vi "Test Zip Methods.vi"() -> ()   [LabVIEW 2016]
uses:
  <userlib>/_OpenG.lib/file/file.llb/Build Path - File Names Array__ogtk.vi
panel:
  out "Numeric":i32=241
  in  "Method":enum16{"MGI", "G", "LV", "7z"}(ring)=enum."7z"
  in  "Table Control":string[][](table)=[["Method", "Size (B)", "Time (s)", "Notes"], ["MGI", "15828699", "20.5822", "Sometimes Errors?"], ["G", "15839557", "5.54458", "Easy to use"], ["LV", "15839557", "4.38332", "Paths cumbersome"], ["7zip", "11000000", "long", "super cumbersome"]]
  out "time (s)":dbl=0.026690200000302866
  out "size (B)":i64
  in  "Root Directory":path=path "C:/user/patrick/git/LV-to-ITX/src/Tests/Example Data/ITX Folder/MNK/SA02836H.20170110/36 - Sweep B - 2"
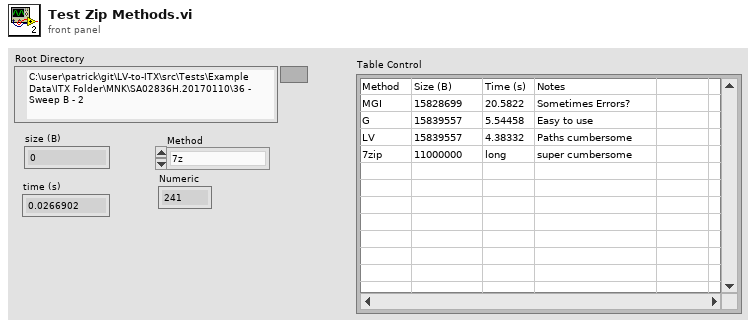
[diagram p1: front panel]
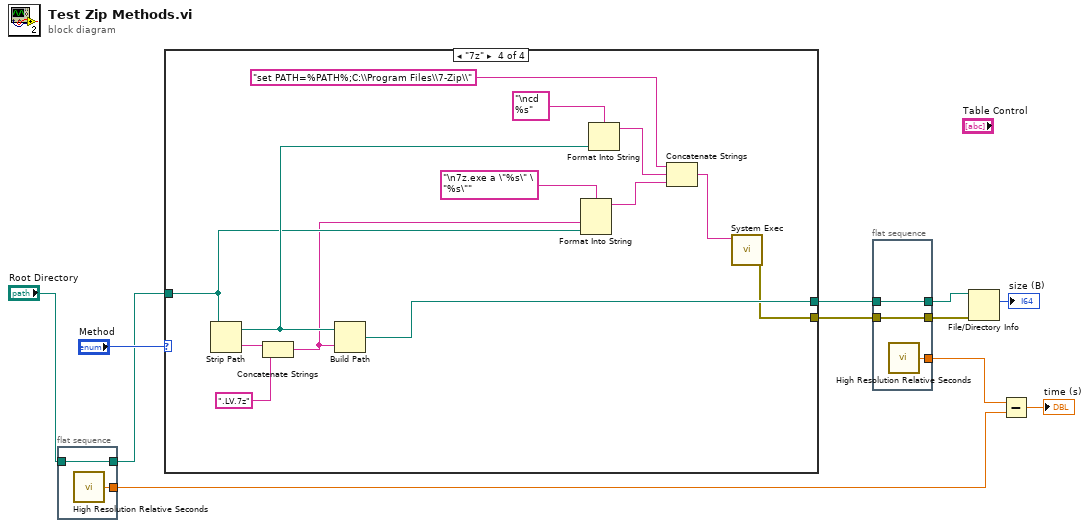
[diagram p0: block diagram]
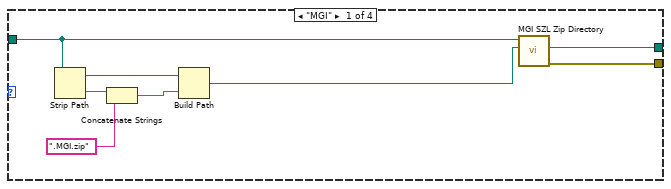
[diagram p2: hidden frame]
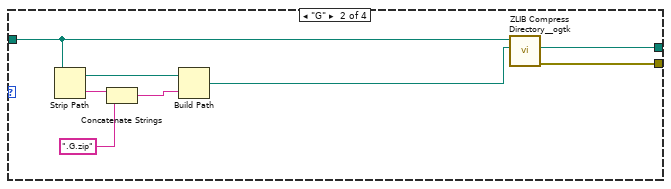
[diagram p3: hidden frame]
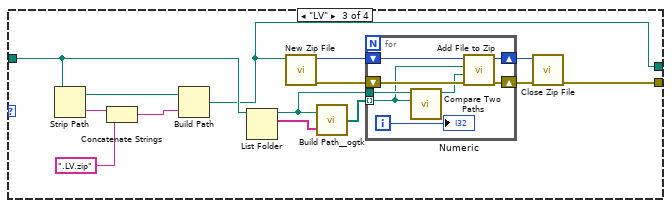
[diagram p4: hidden frame]
diagram:
  n1 = flat-sequence {
    tunnel: [w13] -> w3
    tunnel: [w12] -> w1
    tunnel: "Root Directory" -> [w12]
    frame #0 {
      n2 = call <vilib>:"High Resolution Relative Seconds.vi"() -> ("relative seconds"=w13:dbl)
    }
  }
  n3 = case shown="\"7z\"" "Method" {
    tunnel: w1 -> [w16 w24 w39 w57]
    tunnel: [w15 w23 w32 w54] -> w10
    tunnel: [w14 w22 w33 w53] -> w4
    frame "MGI" {
      n4 = Strip Path(path=w16) -> (stripped path=w19:path, name=w21:string)
      n5 = Concatenate Strings(w21, ".MGI.zip" ("string")) -> (w18:string)
      n6 = Build Path(base path=w19, name or relative path=w18) -> (appended path=w17:path)
      n7 = call <userlib>:"MGI SZL Zip Directory.vi"("Zip File"=w17, "Root Directory"=w16) -> ("Error Out"=w14:errorcluster, "Zip File Out"=w15:path)  [unwired: 7 in, 1 out]
    }
    frame "G" {
      n8 = Strip Path(path=w24) -> (stripped path=w27:path, name=w29:string)
      n9 = Concatenate Strings(w29, ".G.zip" ("string")) -> (w26:string)
      n10 = Build Path(base path=w27, name or relative path=w26) -> (appended path=w25:path)
      n11 = call <userlib>:"ZLIB Compress Directory__ogtk.vi"("archive name (root directory with .zip ending)"=w25, "root directory (file dialog)"=w24) -> ("error out"=w22:errorcluster, "archive name out"=w23:path)  [unwired: 7 in, 1 out]
    }
    frame "LV" {
      n12 = Strip Path(path=w39) -> (stripped path=w41:path, name=w43:string)
      n13 = Concatenate Strings(w43, ".LV.zip" ("string")) -> (w40:string)
      n14 = Build Path(base path=w41, name or relative path=w40) -> (appended path=w32:path)
      n15 = List Folder(path=w39) -> (path out=w30:path, filenames=w38:string[])  [unwired: 3 in, 2 out]
      n16 = call <vilib>:"New Zip File.vi"("target"=w32) -> ("error out"=w35:errorcluster, "zip file out"=w37:i64)  [unwired: 4 in, 1 out]
      n17 = call-poly <userlib>:"Build Path__ogtk.vi"("name or relative path"=w38, "base path"=w30) -> ("appended path"=w31:path[])
      n18 = for {
        tunnel: w30 -> [w46]
        shift-right: [w48] -> w34
        shift-left: w35 -> [w49]
        tunnel: w31 -> [w44] mode=indexing
        shift-right: [w50] -> w36
        shift-left: w37 -> [w51]
        i -> [w45]
        n19 = call <vilib>:"Compare Two Paths.vi"("Path 2"=w44, "Path 1"=w46) -> ("Relative Path from 1 to 2"=w47:path)  [unwired: 6 in, 3 out]
        n20 = call <vilib>:"Add File to Zip.vi"("error in (no error)"=w49, "destination path in zip"=w47, "source file path"=w44, "zip file in"=w51) -> ("error out"=w48:errorcluster, "zip file out"=w50:i64)  [unwired: 6 in]
        "Numeric" <- w45
      }
      n21 = call <vilib>:"Close Zip File.vi"("error in (no error)"=w34, "zip file in"=w36) -> ("error out"=w33:errorcluster)  [unwired: 5 in]
    }
    frame "7z" {
      n22 = Strip Path(path=w57) -> (stripped path=w59:path, name=w64:string)
      n23 = Concatenate Strings(w64, ".LV.7z" ("string")) -> (w56:string)
      n24 = Build Path(base path=w59, name or relative path=w56) -> (appended path=w54:path)
      n25 = Format Into String(format string="\n7z.exe a \"%s\" \"%s\"" ("Name of target (My Computer)"), w56, w57) -> (resulting string=w55:string)  [unwired: 2 in, 1 out]
      n26 = Format Into String(format string="\ncd %s" ("Name of target (My Computer)"), w59) -> (resulting string=w60:string)  [unwired: 2 in, 1 out]
      n27 = Concatenate Strings("set PATH=%PATH%;C:\\Program Files\\7-Zip\\" ("Name of target (My Computer)"), w60, w55) -> (w52:string)
      n28 = call <vilib>:"System Exec.vi"("command line"=w52) -> ("error out"=w53:errorcluster)  [unwired: 7 in, 3 out]
    }
  }
  n29 = flat-sequence {
    tunnel: [w67] -> w11
    tunnel: w10 -> [w66]
    tunnel: [w66] -> w9
    tunnel: [w65] -> w5
    tunnel: w4 -> [w65]
    frame #0 {
      n30 = call <vilib>:"High Resolution Relative Seconds.vi"() -> ("relative seconds"=w67:dbl)
    }
  }
  n31 = File/Directory Info(path=w9, error in=w5) -> (size=→"size (B)":i64)  [unwired: 6 out]
  n32 = Subtract(x=w11, y=w3) -> (x-y=→"time (s)":dbl)
